vi "Init_Write_CMD_Buffer.vi"(8 "error in (no error)":errorcluster, 11 "DeviceNum":i32) -> (0 "error out":errorcluster)   [LabVIEW 2020, in "LabSCADA.lvlib"]
uses:
  LabSCADA.lvlib
  DynamicIOCMD.lvlib
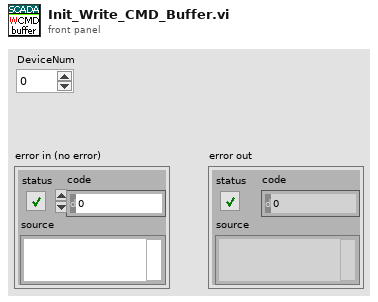
[diagram p1: front panel]
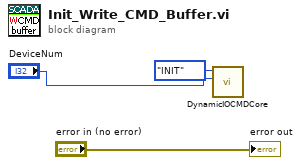
[diagram p0: block diagram]
diagram:
  n1 = call "DynamicIOCMDCore.vi"("DeviceIndex"="DeviceNum", "Function"=enum16{"INIT", "NEW", "GET"}."INIT") -> ()  [unwired: 8 in, 2 out]
  "error out" <- "error in (no error)"
